vi "Close.vi"(8 "error in (no error)":errorcluster, 11 "VIEW in":refnum<class "VIEW.lvclass">) -> (0 "error out":errorcluster, 3 "VIEW out":refnum<class "VIEW.lvclass">)   [LabVIEW 2013, in "VIEW.lvclass"]
uses:
  VIEW.lvclass
  VIEW.lvclass/VIEW.ctl
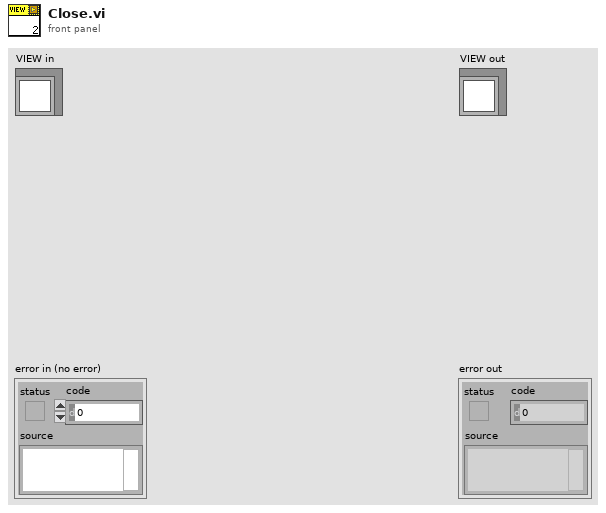
[diagram p1: front panel]
types:
  T1 = cluster{"CtlRef":refnum<vi>, "Name":string, "ClassName":string}[]
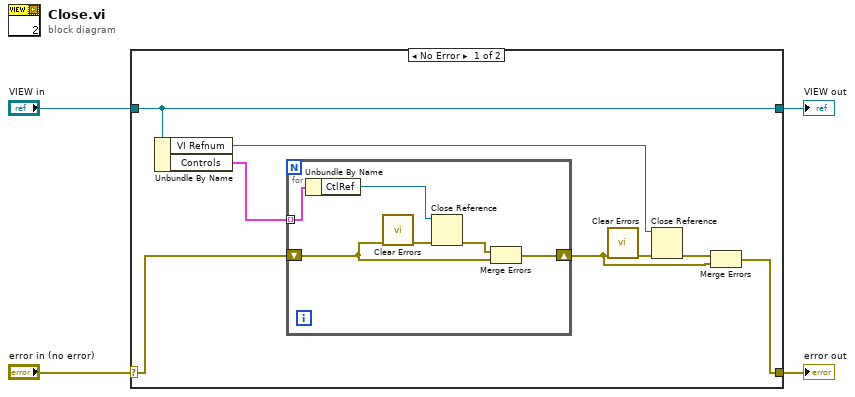
[diagram p0: block diagram]
diagram:
  n1 = case shown="No Error" "error in (no error)" {
    selector: "error in (no error)" -> [w10 w20]
    tunnel: [w6 w20] -> w3
    tunnel: [w12 w19] -> w1
    tunnel: "VIEW in" -> [w12 w19]
    frame No Error {
      n2 = Unbundle By Name(w12) -> ("VI Refnum"=w5:refnum<vi>, "Controls"=w11:T1)
      n3 = for {
        tunnel: w11 -> [w18] mode=indexing
        shift-right: [w13] -> w7
        shift-left: w10 -> [w14]
        n4 = Unbundle By Name(w18) -> ("CtlRef"=w17:refnum<vi>)
        n5 = call <vilib>:"Clear Errors.vi"("error in (no error)"=w14) -> ("error out"=w16:errorcluster)  [unwired: 6 in]
        n6 = Close Reference(reference=w17, error in (no error)=w16) -> (error out=w15:errorcluster)
        n7 = Merge Errors(w15, w14) -> (w13:errorcluster)
      }
      n8 = call <vilib>:"Clear Errors.vi"("error in (no error)"=w7) -> ("error out"=w9:errorcluster)  [unwired: 6 in]
      n9 = Close Reference(reference=w5, error in (no error)=w9) -> (error out=w8:errorcluster)
      n10 = Merge Errors(w8, w7) -> (w6:errorcluster)
    }
    frame Error {
    }
  }
  "error out" <- w3
  "VIEW out" <- w1
